vi "Instrument.AML Example.vi"   [LabVIEW 2019]
uses:
  Instrument.AML.GetAll--Cluster.ctl
  <userlib>/LevyLab/LV-Data/LV-Data.PG/LV-Data.PGSQL.lvclass
panel:
  # "Open Block Diagram"
types:
  T1 = typedef "Instrument.AML.GetAll--Cluster.ctl" = cluster{"IG Pressure (mbar)":dbl, "Pirani 1 Pressure (mbar)":dbl, "Pirani 2 Pressure (mbar)":dbl, "Emission Current (A)":dbl, "Trip A Pressure (mbar)":dbl, "Trip B Pressure (mbar)":dbl, "Trip C Pressure (mbar)":dbl, "Trip D Pressure (mbar)":dbl, "Instrument Status":string, "Fault":string, "Trip A Association":string, "Trip B Association":string, "Trip C Association":string, "Trip D Association":string, "Relay A":string, "Relay B":string, "Relay C":string, "Relay D":string}
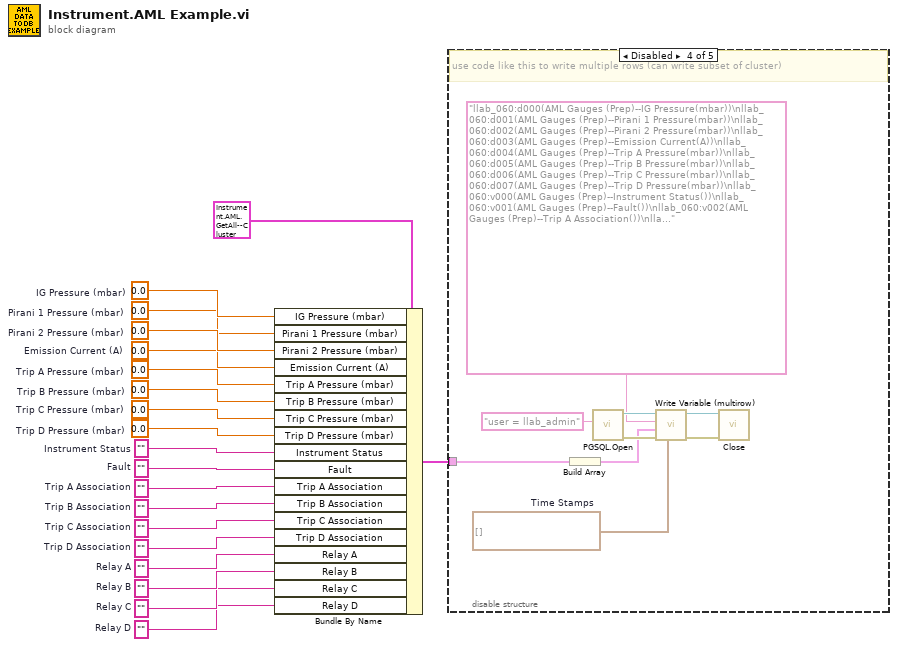
[diagram p0: block diagram]
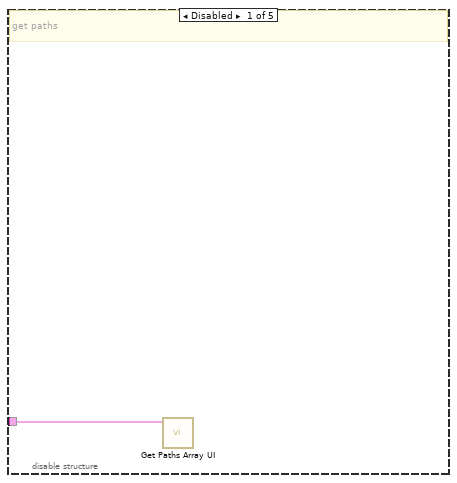
[diagram p2: hidden frame]
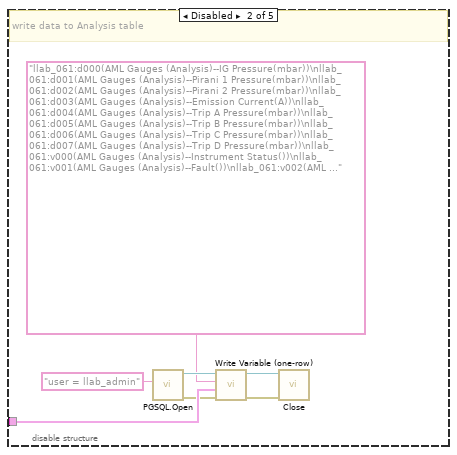
[diagram p3: hidden frame]
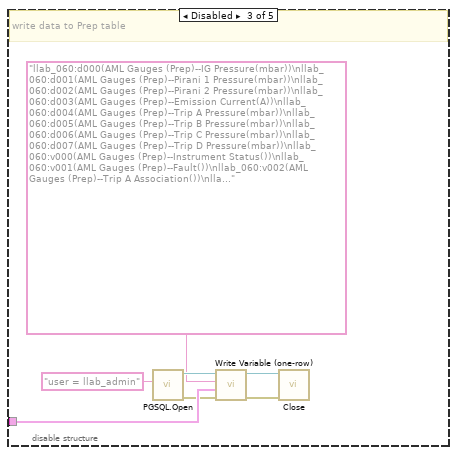
[diagram p4: hidden frame]
diagram:
  w5 = ""  # Relay D
  w6 = ""  # Relay C
  w7 = ""  # Relay B
  w8 = ""  # Relay A
  w9 = ""  # Trip D Association
  w10 = ""  # Trip C Association
  w11 = ""  # Trip B Association
  w12 = ""  # Trip A Association
  w13 = ""  # Fault
  w14 = ""  # Instrument Status
  w15 = 0.0  # Trip D Pressure (mbar)
  w16 = 0.0  # Trip C Pressure (mbar)
  w17 = 0.0  # Trip B Pressure (mbar)
  w18 = 0.0  # Trip A Pressure (mbar)
  w19 = 0.0  # Emission Current (A)
  w20 = 0.0  # Pirani 2 Pressure (mbar)
  w3 = 0.0  # Pirani 1 Pressure (mbar)
  w4 = 0.0  # IG Pressure (mbar)
  n1 = Bundle By Name(cluster=T1 {"IG Pressure (mbar)"=0.0, "Pirani 1 Pressure (mbar)"=0.0, "Pirani 2 Pressure (mbar)"=0.0, "Emission Current (A)"=0.0, "Trip A Pressure (mbar)"=0.0, "Trip B Pressure (mbar)"=0.0, "Trip C Pressure (mbar)"=0.0, "Trip D Pressure (mbar)"=0.0, "Instrument Status"="", "Fault"="", "Trip A Association"="", "Trip B Association"="", "Trip C Association"="", "Trip D Association"="", "Relay A"="", "Relay B"="", "Relay C"="", "Relay D"=""}, "IG Pressure (mbar)"=w4, "Pirani 1 Pressure (mbar)"=w3, "Pirani 2 Pressure (mbar)"=w20, "Emission Current (A)"=w19, "Trip A Pressure (mbar)"=w18, "Trip B Pressure (mbar)"=w17, "Trip C Pressure (mbar)"=w16, "Trip D Pressure (mbar)"=w15, "Instrument Status"=w14, "Fault"=w13, "Trip A Association"=w12, "Trip B Association"=w11, "Trip C Association"=w10, "Trip D Association"=w9, "Relay A"=w8, "Relay B"=w7, "Relay C"=w6, "Relay D"=w5) -> (w1:T1)
  n2 = disable-structure shown="Disabled" {
    disable-tunnel: w1 -> [w21 w27 w34 w43 _]
    frame Disabled {
      # "get paths"
      n3 = call <userlib>:"Get Paths Array UI.vi"("Data"=w21) -> ()  [unwired: 9 in, 2 out]
    }
    frame Disabled {
      # "write data to Analysis table"
      n4 = call <userlib>:"PGSQL.Open.vi"("Connection String"="user = llab_admin") -> ("error out"=w26:errorcluster, "Data.PG out"=w25:refnum<class "LV-Data.PGSQL.lvclass">)  [unwired: 9 in]
      n5 = call <userlib>:"Write Variable (one-row).vi"("error in (no error)"=w26, "Data"=w27, "variable"="llab_061:d000(AML Gauges (Analysis)--IG Pressure(mbar))\nllab_061:d001(AML Gauges (Analysis)--Pirani 1 Pressure(mbar))\nllab_061:d002(AML Gauges (Analysis)--Pirani 2 Pressure(mbar))\nllab_061:d003(AML Gauges (Analysis)--Emission Current(A))\nllab_061:d004(AML Gauges (Analysis)--Trip A Pressure(mbar))\nllab_061:d005(AML Gauges (Analysis)--Trip B Pressure(mbar))\nllab_061:d006(AML Gauges (Analysis)--Trip C Pressure(mbar))\nllab_061:d007(AML Gauges (Analysis)--Trip D Pressure(mbar))\nllab_061:v000(AML Gauges (Analysis)--Instrument Status())\nllab_061:v001(AML Gauges (Analysis)--Fault())\nllab_061:v002(AML Gauges (Analysis)--Trip A Association())\nllab_061:v003(AML Gauges (Analysis)--Trip B Association())\nllab_061:v004(AML Gauges (Analysis)--Trip C Association())\nllab_061:v005(AML Gauges (Analysis)--Trip D Association())\nllab_061:v006(AML Gauges (Analysis)--Relay A())\nllab_061:v007(AML Gauges (Analysis)--Relay B())\nllab_061:v008(AML Gauges (Analysis)--Relay C())\nllab_061:v009(AML Gauges (Analysis)--Relay D())", "Data.PG in"=w25) -> ("error out"=w22:errorcluster, "Data.PG out"=w23:refnum<class "LV-Data.PGSQL.lvclass">)  [unwired: 4 in, 2 out]
      n6 = call-dynamic "Close.vi"("error in (no error)"=w22, "Data.PG in"=w23) -> ()  [unwired: 8 in, 2 out]
    }
    frame Disabled {
      # "write data to Prep table"
      n7 = call <userlib>:"PGSQL.Open.vi"("Connection String"="user = llab_admin") -> ("error out"=w33:errorcluster, "Data.PG out"=w32:refnum<class "LV-Data.PGSQL.lvclass">)  [unwired: 9 in]
      n8 = call <userlib>:"Write Variable (one-row).vi"("error in (no error)"=w33, "Data"=w34, "variable"="llab_060:d000(AML Gauges (Prep)--IG Pressure(mbar))\nllab_060:d001(AML Gauges (Prep)--Pirani 1 Pressure(mbar))\nllab_060:d002(AML Gauges (Prep)--Pirani 2 Pressure(mbar))\nllab_060:d003(AML Gauges (Prep)--Emission Current(A))\nllab_060:d004(AML Gauges (Prep)--Trip A Pressure(mbar))\nllab_060:d005(AML Gauges (Prep)--Trip B Pressure(mbar))\nllab_060:d006(AML Gauges (Prep)--Trip C Pressure(mbar))\nllab_060:d007(AML Gauges (Prep)--Trip D Pressure(mbar))\nllab_060:v000(AML Gauges (Prep)--Instrument Status())\nllab_060:v001(AML Gauges (Prep)--Fault())\nllab_060:v002(AML Gauges (Prep)--Trip A Association())\nllab_060:v003(AML Gauges (Prep)--Trip B Association())\nllab_060:v004(AML Gauges (Prep)--Trip C Association())\nllab_060:v005(AML Gauges (Prep)--Trip D Association())\nllab_060:v006(AML Gauges (Prep)--Relay A())\nllab_060:v007(AML Gauges (Prep)--Relay B())\nllab_060:v008(AML Gauges (Prep)--Relay C())\nllab_060:v009(AML Gauges (Prep)--Relay D())", "Data.PG in"=w32) -> ("error out"=w29:errorcluster, "Data.PG out"=w30:refnum<class "LV-Data.PGSQL.lvclass">)  [unwired: 4 in, 2 out]
      n9 = call-dynamic "Close.vi"("error in (no error)"=w29, "Data.PG in"=w30) -> ()  [unwired: 8 in, 2 out]
    }
    frame Disabled {
      w36 = timestamp[] []  # Time Stamps
      # "use code like this to write multiple rows (can write subset of cluster)"
      n10 = Build Array(w43) -> (w37:T1[])
      n11 = call <userlib>:"PGSQL.Open.vi"("Connection String"="user = llab_admin") -> ("error out"=w42:errorcluster, "Data.PG out"=w41:refnum<class "LV-Data.PGSQL.lvclass">)  [unwired: 9 in]
      n12 = call <userlib>:"Write Variable (multirow).vi"("Time Stamps"=w36, "error in (no error)"=w42, "Data"=w37, "Path(s)"="llab_060:d000(AML Gauges (Prep)--IG Pressure(mbar))\nllab_060:d001(AML Gauges (Prep)--Pirani 1 Pressure(mbar))\nllab_060:d002(AML Gauges (Prep)--Pirani 2 Pressure(mbar))\nllab_060:d003(AML Gauges (Prep)--Emission Current(A))\nllab_060:d004(AML Gauges (Prep)--Trip A Pressure(mbar))\nllab_060:d005(AML Gauges (Prep)--Trip B Pressure(mbar))\nllab_060:d006(AML Gauges (Prep)--Trip C Pressure(mbar))\nllab_060:d007(AML Gauges (Prep)--Trip D Pressure(mbar))\nllab_060:v000(AML Gauges (Prep)--Instrument Status())\nllab_060:v001(AML Gauges (Prep)--Fault())\nllab_060:v002(AML Gauges (Prep)--Trip A Association())\nllab_060:v003(AML Gauges (Prep)--Trip B Association())\nllab_060:v004(AML Gauges (Prep)--Trip C Association())\nllab_060:v005(AML Gauges (Prep)--Trip D Association())\nllab_060:v006(AML Gauges (Prep)--Relay A())\nllab_060:v007(AML Gauges (Prep)--Relay B())\nllab_060:v008(AML Gauges (Prep)--Relay C())\nllab_060:v009(AML Gauges (Prep)--Relay D())", "Data.PG in"=w41) -> ("error out"=w38:errorcluster, "Data.PG out"=w39:refnum<class "LV-Data.PGSQL.lvclass">)  [unwired: 3 in, 2 out]
      n13 = call-dynamic "Close.vi"("error in (no error)"=w38, "Data.PG in"=w39) -> ()  [unwired: 8 in, 2 out]
    }
    frame Enabled {
    }
  }
